vi "hcam_environment_monitor.vi"() -> ()   [LabVIEW 2020]
uses:
  <vilib>/Instr/_visa.llb/VISA Configure Serial Port (Instr).vi
panel:
  in  "INT 2":u8 caption="Brightness"
  in  "SEND INT 2":bool caption="Boolean"
  out "Humidity 2":string caption="Humidity"
  in  "Start 2":timestamp caption="Day Start" format="%<%H:%M>T"
  in  "End 2":timestamp caption="Day End" format="%<%H:%M>T"
  in  "SEND LED 2":bool caption="Boolean"
  in  "SEND RTC 2":bool caption="Boolean"
  in  "Color Box 2":u32(colorbox) caption="Color"
  out "Temp 2":string caption="Temp"
  in  "End":timestamp caption="Day End" format="%<%H:%M>T"
  in  "Start":timestamp caption="Day Start" format="%<%H:%M>T"
  in  "SEND LED":bool caption="Boolean"
  in  "Color Box":u32(colorbox) caption="Color"
  in  "SEND RTC":bool caption="Boolean"
  out "Humidity":string
  out "Temp":string
  in  "SEND INT":bool caption="Boolean"
  in  "INT":u8 caption="Brightness"
  out "Connected":bool
  out "Response":string
  in  "CONNECTION":bool
  out "Bytes Read":u32
  in  "VISA Resource":refnum<visa-resource-name>="COM1"
  # "--- Box 1 ---"
  # "--- Box 2 ---"
  # "Auto LED Timer"
  # "Auto LED Timer"
  # "Manual Color Control"
  # "Climate Readings"
  # "Manual Color Control"
  # "Climate Readings"
  # "Serial Monitor"
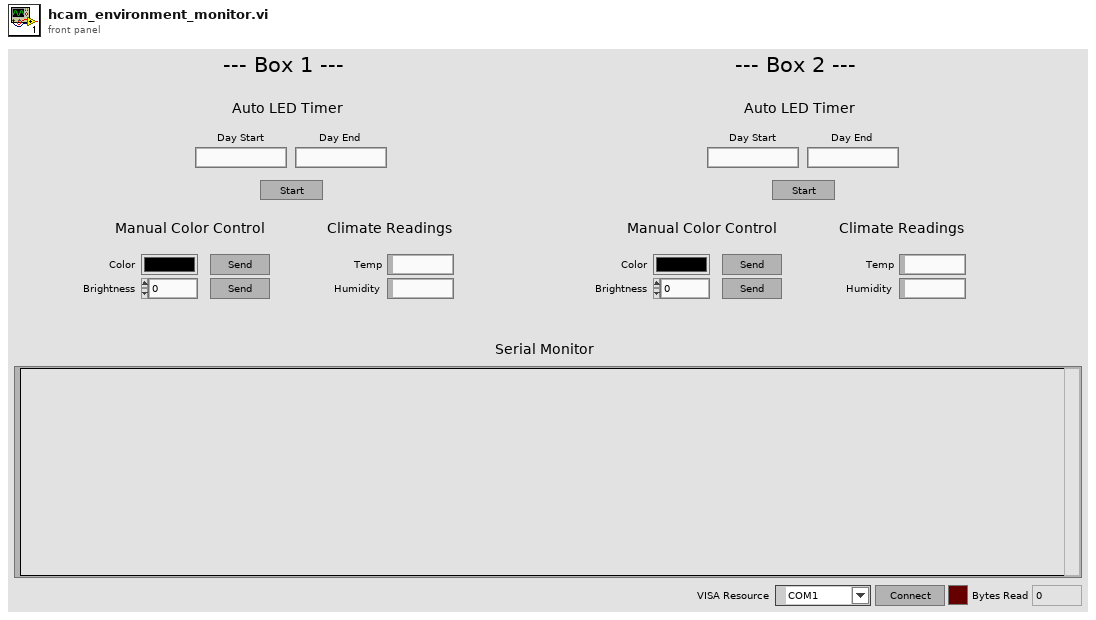
[diagram p1: front panel]
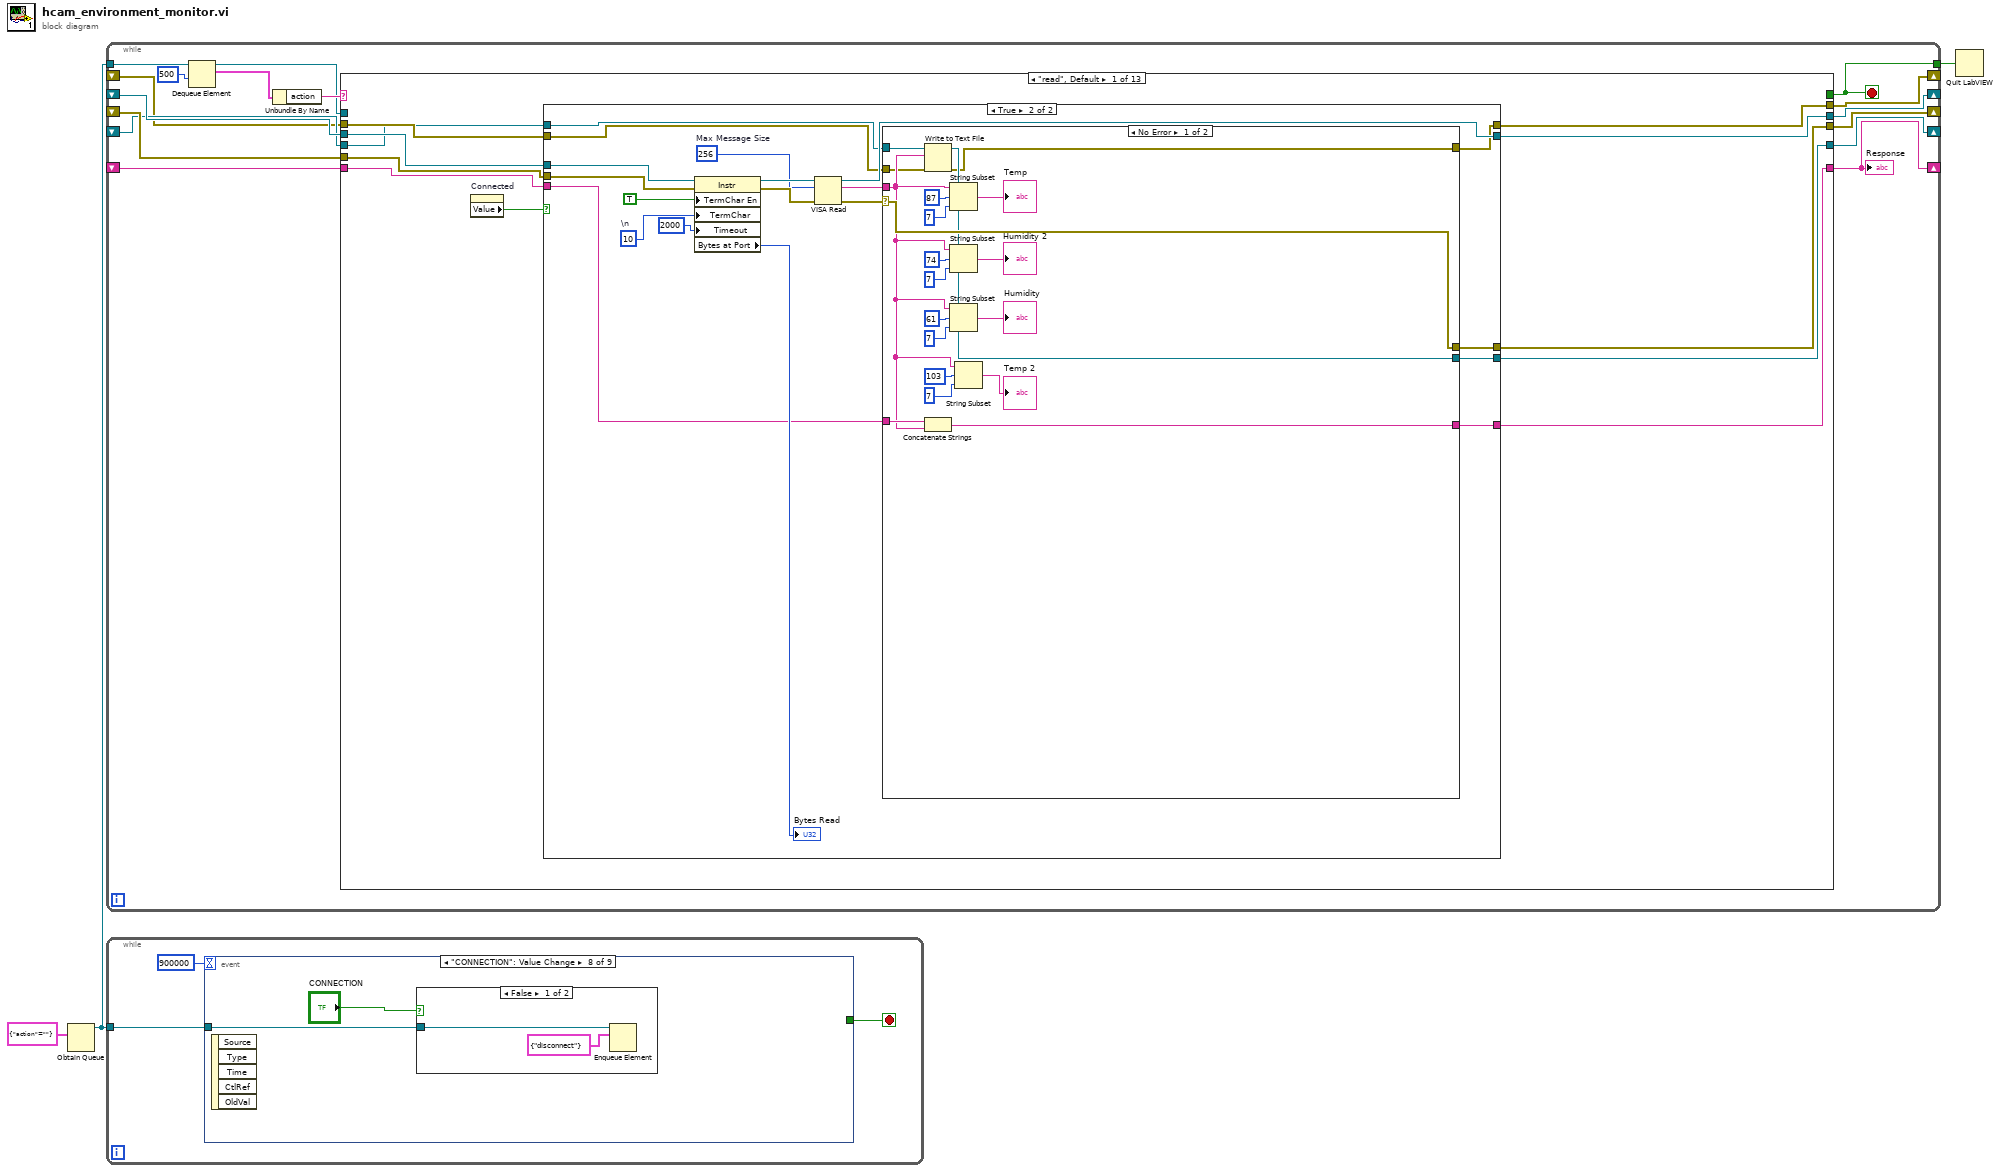
[diagram p0: block diagram]
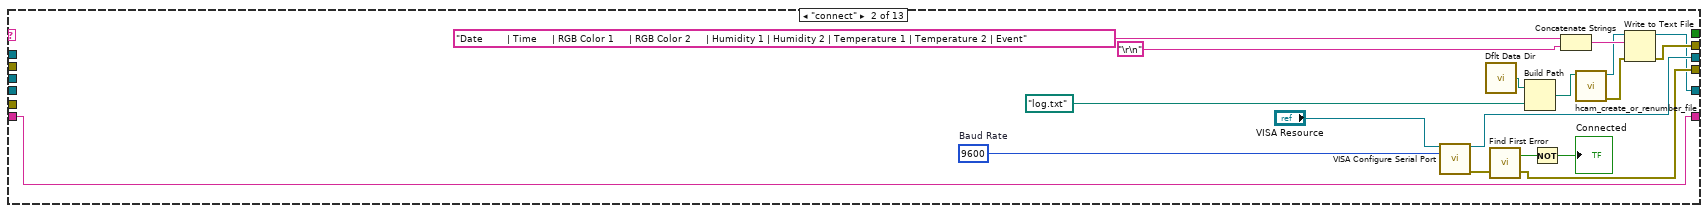
[diagram p4: hidden frame]
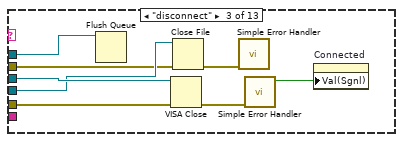
[diagram p5: hidden frame]
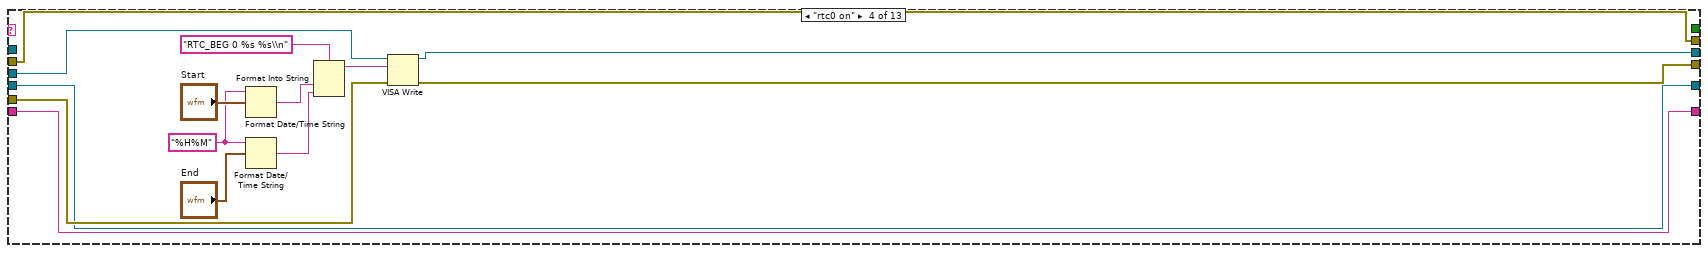
[diagram p6: hidden frame]
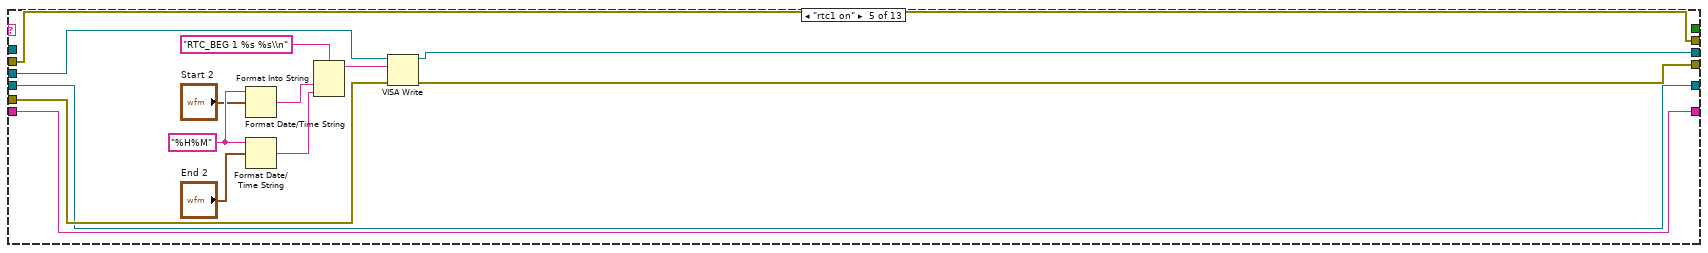
[diagram p7: hidden frame]
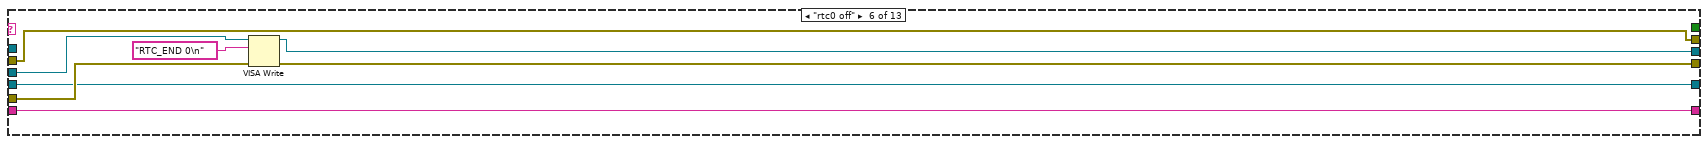
[diagram p8: hidden frame]
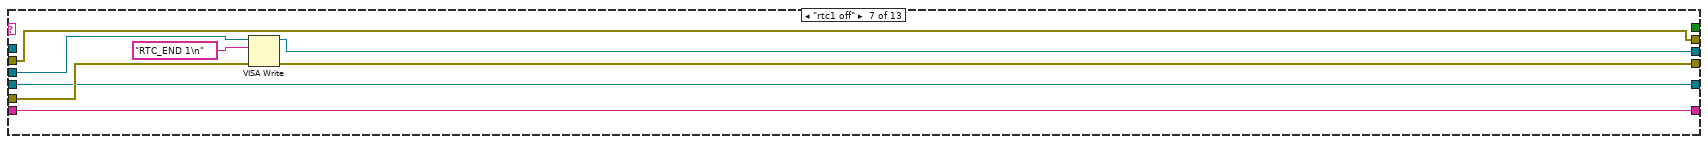
[diagram p9: hidden frame]
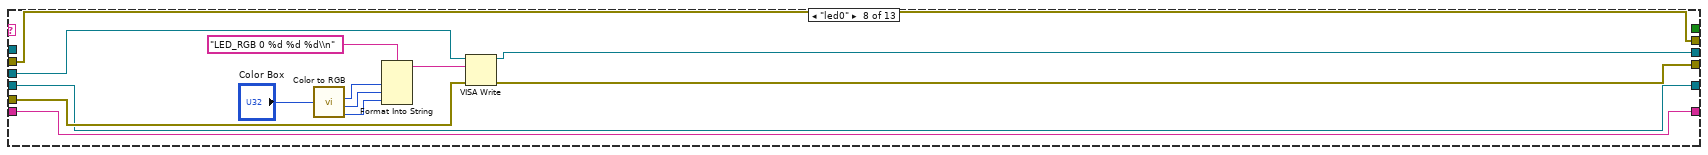
[diagram p10: hidden frame]
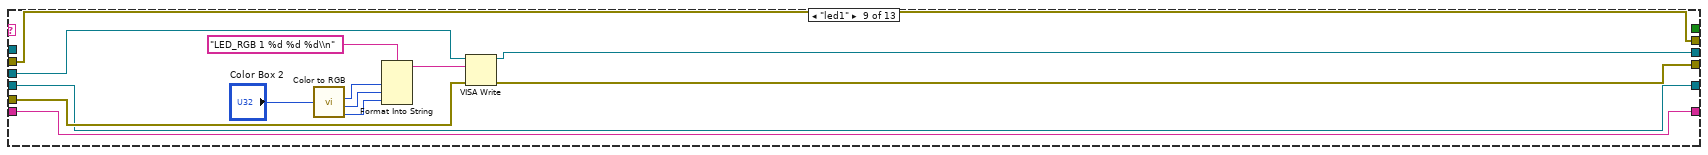
[diagram p11: hidden frame]
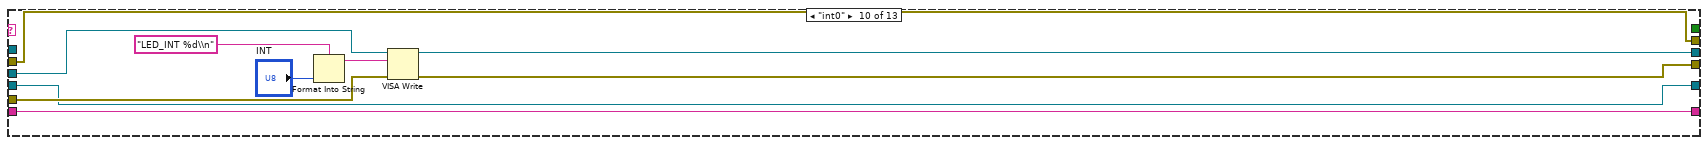
[diagram p12: hidden frame]
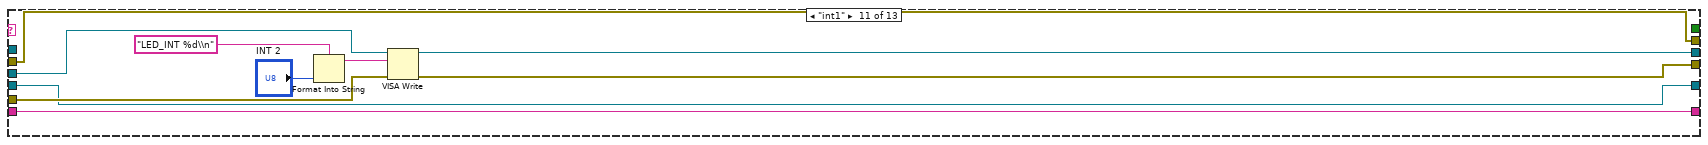
[diagram p13: hidden frame]
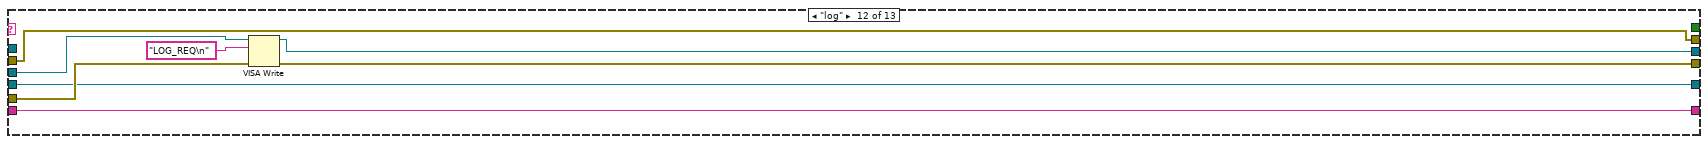
[diagram p14: hidden frame]
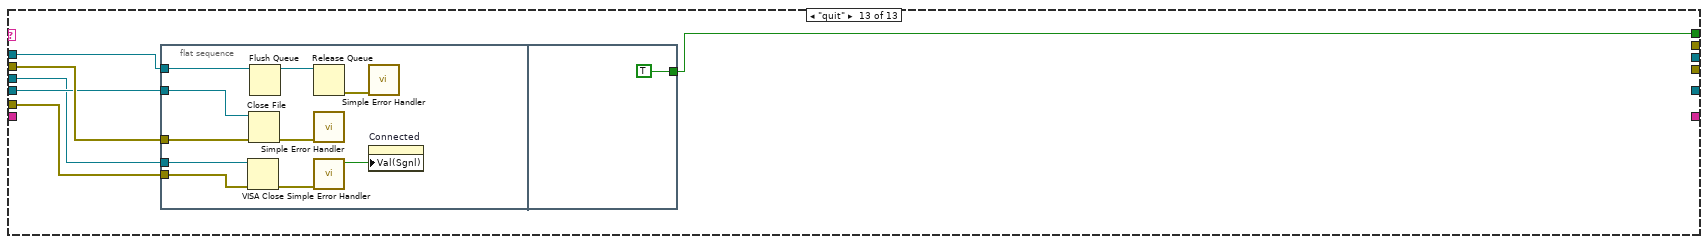
[diagram p15: hidden frame]
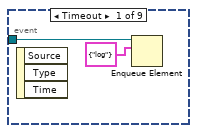
[diagram p16: hidden frame]
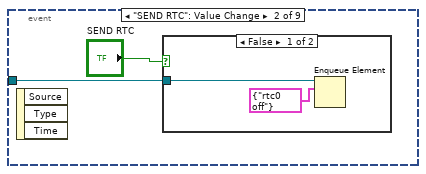
[diagram p17: hidden frame]
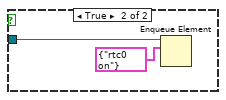
[diagram p18: hidden frame]
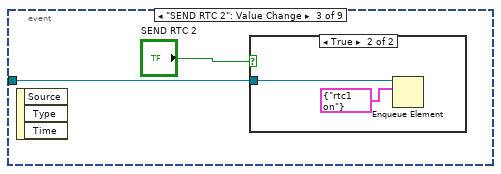
[diagram p19: hidden frame]
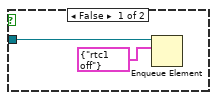
[diagram p20: hidden frame]
diagram:
  n1 = Obtain Queue(element data type=cluster{"action":string} {"action"=""}) -> (queue out=w2:refnum<queue>)  [unwired: 4 in, 2 out]
  n2 = while {
    tunnel: w2 -> [w19]
    shift-right: [w14] -> _
    shift-left: _ -> [w13]
    shift-right: [w12] -> _
    shift-left: _ -> [w11]
    shift-right: [w9] -> _
    shift-left: _ -> [w10]
    shift-right: [w6] -> _
    shift-left: _ -> [w8]
    shift-right: [w5] -> _
    shift-left: _ -> [w7]
    tunnel: [w4] -> w1
    stop <- w4 stop-if-true
    n3 = Dequeue Element(queue=w19, timeout in ms (-1)=500) -> (queue out=w15:refnum<queue>, element=w17:cluster{"action":string})  [unwired: 1 in, 2 out]
    n4 = Unbundle By Name(w17) -> ("action"=w16:string)
    n5 = case shown="\"read\", Default" w16 {
      tunnel: w15 -> [_ _ w95 _ _ _ _ _ _ _ _ _ w200]
      tunnel: [w24 w88 _ w104 w119 w133 w141 w152 w165 w175 w185 w192 _] -> w14
      tunnel: w13 -> [w30 _ w98 w105 w118 w134 w142 w153 w166 w176 w186 w193 w198]
      tunnel: [w28 w86 _ w102 w116 w131 w139 w150 w163 w172 w183 w194 _] -> w12
      tunnel: w11 -> [w29 _ w96 w103 w117 w132 w140 w151 w164 w173 w184 w195 w199]
      tunnel: [w26 w83 _ w101 w115 w130 w138 w149 w162 w171 w182 w196 _] -> w9
      tunnel: w10 -> [w27 w83 _ w101 w115 w130 w138 w149 w162 w171 w182 w196 _]
      tunnel: [w21 w79 _ w100 w114 w128 w136 w144 w157 w170 w180 w190 _] -> w6
      tunnel: [w20 w80 _ w99 w113 w127 w135 w143 w156 w169 w179 w189 _] -> w5
      tunnel: w8 -> [w22 _ w93 w100 w114 w128 w136 w144 w157 w170 w180 w190 w201]
      tunnel: w7 -> [w23 _ w92 w99 w113 w127 w135 w143 w156 w169 w179 w189 w202]
      tunnel: [_ _ _ _ _ _ _ _ _ _ _ _ w197] -> w4
      frame "read", Default {
        n6 = property on="Connected" class="Bool (strict)"() -> ("Value"=w25:bool)  [unwired: 2 in, 2 out]
        n7 = case shown="True" w25 {
          tunnel: w30 -> [_ w42]
          tunnel: w29 -> [_ w41]
          tunnel: [_ w36] -> w28
          tunnel: w27 -> [_ w38]
          tunnel: [_ w35] -> w26
          tunnel: [_ w40] -> w24
          tunnel: [_ w31] -> w20
          tunnel: [_ w32] -> w21
          tunnel: w23 -> [_ w34]
          tunnel: w22 -> [_ w33]
          frame False {
          }
          frame True {
            w46 = u32 256  # Max Message Size
            w44 = u8 10  # \n
            n8 = property class="Instr"(reference=w42, error in=w41, "TermChar En"=TRUE ("Message Based Settings:Termination Character Enable"), "TermChar"=w44, "Timeout"=u32 2000 ("General Settings:Timeout Value")) -> (reference out=w49:refnum<visa-resource-name>, error out=w48:errorcluster, "Bytes at Port"=→"Bytes Read":u32)
            n9 = VISA Read(VISA resource name=w49, byte count=w46, error in (no error)=w48) -> (VISA resource name out=w40:refnum<visa-resource-name>, read buffer=w37:string, error out=w39:errorcluster)  [unwired: 1 out]
            n10 = case shown="No Error" w39 {
              selector: w39 -> [w68 _]
              tunnel: w38 -> [w69 w72]
              tunnel: w37 -> [w54 _]
              tunnel: [w67 w72] -> w35
              tunnel: [w68 _] -> w36
              tunnel: w34 -> [w53 w71]
              tunnel: w33 -> [w52 w70]
              tunnel: [w51 w70] -> w32
              tunnel: [w50 w71] -> w31
              frame No Error {
                n11 = Write to Text File(file (use dialog)=w52, text=w54, error in=w53) -> (refnum out=w51:refnum<file>, error out=w50:errorcluster)  [unwired: 1 in, 1 out]
                n12 = Concatenate Strings(w69, w54) -> (w67:string)
                n13 = String Subset(string=w54, offset (0)=87, length (rest)=7) -> (substring=→"Temp":string)
                n14 = String Subset(string=w54, offset (0)=74, length (rest)=7) -> (substring=→"Humidity 2":string)
                n15 = String Subset(string=w54, offset (0)=61, length (rest)=7) -> (substring=→"Humidity":string)
                n16 = String Subset(string=w54, offset (0)=103, length (rest)=7) -> (substring=→"Temp 2":string)
              }
              frame Error {
              }
            }
          }
        }
      }
      frame "connect" {
        w89 = u32 9600  # Baud Rate
        n17 = call-poly "VISA Configure Serial Port"("VISA resource name"="VISA Resource", "baud rate (9600)"=w89) -> ("VISA resource name out"=w88:refnum<visa-resource-name>, "error out"=w87:errorcluster)  [unwired: 7 in, 5 out]
        n18 = call <vilib>:"Dflt Data Dir.vi"() -> ("App:Default Data Directory"=w82:path)
        n19 = call <vilib>:"Find First Error.vi"("error in (no error)"=w87) -> ("error out"=w86:errorcluster, "error?"=w85:bool)  [unwired: 3 in]
        n20 = Build Path(base path=w82, name or relative path=path "log.txt" ("default name")) -> (appended path=w75:path)
        n21 = Not(x=w85) -> (.not. x?=→"Connected":bool)
        n22 = Concatenate Strings("Date        | Time     | RGB Color 1     | RGB Color 2     | Humidity 1 | Humidity 2 | Temperature 1 | Temperature 2 | Event", "\r\n") -> (w76:string)
        n23 = call "hcam_create_or_renumber_file.vi"("file path"=w75) -> ("error out"=w73:errorcluster, "refnum out"=w74:refnum<file>)  [unwired: 9 in]
        n24 = Write to Text File(file (use dialog)=w74, text=w76, error in=w73) -> (refnum out=w79:refnum<file>, error out=w80:errorcluster)  [unwired: 1 in, 1 out]
      }
      frame "disconnect" {
        n25 = Flush Queue(queue=w95) -> ()  [unwired: 1 in, 3 out]
        n26 = VISA Close(VISA resource name=w98, error in (no error)=w96) -> (error out=w97:errorcluster)
        n27 = Close File(refnum=w93, error in=w92) -> (error out=w91:errorcluster)  [unwired: 1 out]
        n28 = call <vilib>:"Simple Error Handler.vi"("error in (no error)"=w91) -> ()  [unwired: 4 in, 5 out]
        n29 = call <vilib>:"Simple Error Handler.vi"("error in (no error)"=w97) -> ("error?"=w94:bool)  [unwired: 1 in, 7 out]
        n30 = property on="Connected" class="Bool (strict)"("Val(Sgnl)"=w94) -> ()  [unwired: 2 in, 2 out]
      }
      frame "rtc0 on" {
        w106 = "%H%M"
        n31 = Format Date/Time String(time format string (%c)=w106, seconds (now)="Start") -> (date/time string=w112:string)  [unwired: 1 in]
        n32 = Format Date/Time String(time format string (%c)=w106, seconds (now)="End") -> (date/time string=w111:string)  [unwired: 1 in]
        n33 = Format Into String(format string="RTC_BEG 0 %s %s\\n", w112, w111) -> (resulting string=w108:string)  [unwired: 2 in, 1 out]
        n34 = VISA Write(VISA resource name=w105, write buffer=w108, error in (no error)=w103) -> (VISA resource name out=w104:refnum<visa-resource-name>, error out=w102:errorcluster)  [unwired: 1 out]
      }
      frame "rtc1 on" {
        w124 = "%H%M"
        n35 = Format Date/Time String(time format string (%c)=w124, seconds (now)="Start 2") -> (date/time string=w122:string)  [unwired: 1 in]
        n36 = Format Date/Time String(time format string (%c)=w124, seconds (now)="End 2") -> (date/time string=w123:string)  [unwired: 1 in]
        n37 = Format Into String(format string="RTC_BEG 1 %s %s\\n", w122, w123) -> (resulting string=w125:string)  [unwired: 2 in, 1 out]
        n38 = VISA Write(VISA resource name=w118, write buffer=w125, error in (no error)=w117) -> (VISA resource name out=w119:refnum<visa-resource-name>, error out=w116:errorcluster)  [unwired: 1 out]
      }
      frame "rtc0 off" {
        n39 = VISA Write(VISA resource name=w134, write buffer="RTC_END 0\n" ("format string"), error in (no error)=w132) -> (VISA resource name out=w133:refnum<visa-resource-name>, error out=w131:errorcluster)  [unwired: 1 out]
      }
      frame "rtc1 off" {
        n40 = VISA Write(VISA resource name=w142, write buffer="RTC_END 1\n" ("format string"), error in (no error)=w140) -> (VISA resource name out=w141:refnum<visa-resource-name>, error out=w139:errorcluster)  [unwired: 1 out]
      }
      frame "led0" {
        n41 = call <vilib>:"Color to RGB.vi"("Color"="Color Box") -> ("R"=w147:u8, "G"=w146:u8, "B"=w145:u8)  [unwired: 1 out]
        n42 = Format Into String(format string="LED_RGB 0 %d %d %d\\n", w147, w146, w145) -> (resulting string=w154:string)  [unwired: 2 in, 1 out]
        n43 = VISA Write(VISA resource name=w153, write buffer=w154, error in (no error)=w151) -> (VISA resource name out=w152:refnum<visa-resource-name>, error out=w150:errorcluster)  [unwired: 1 out]
      }
      frame "led1" {
        n44 = call <vilib>:"Color to RGB.vi"("Color"="Color Box 2") -> ("R"=w160:u8, "G"=w159:u8, "B"=w158:u8)  [unwired: 1 out]
        n45 = Format Into String(format string="LED_RGB 1 %d %d %d\\n", w160, w159, w158) -> (resulting string=w167:string)  [unwired: 2 in, 1 out]
        n46 = VISA Write(VISA resource name=w166, write buffer=w167, error in (no error)=w164) -> (VISA resource name out=w165:refnum<visa-resource-name>, error out=w163:errorcluster)  [unwired: 1 out]
      }
      frame "int0" {
        n47 = Format Into String(format string="LED_INT %d\\n", "INT") -> (resulting string=w177:string)  [unwired: 2 in, 1 out]
        n48 = VISA Write(VISA resource name=w176, write buffer=w177, error in (no error)=w173) -> (VISA resource name out=w175:refnum<visa-resource-name>, error out=w172:errorcluster)  [unwired: 1 out]
      }
      frame "int1" {
        n49 = Format Into String(format string="LED_INT %d\\n", "INT 2") -> (resulting string=w187:string)  [unwired: 2 in, 1 out]
        n50 = VISA Write(VISA resource name=w186, write buffer=w187, error in (no error)=w184) -> (VISA resource name out=w185:refnum<visa-resource-name>, error out=w183:errorcluster)  [unwired: 1 out]
      }
      frame "log" {
        n51 = VISA Write(VISA resource name=w193, write buffer="LOG_REQ\n" ("format string"), error in (no error)=w195) -> (VISA resource name out=w192:refnum<visa-resource-name>, error out=w194:errorcluster)  [unwired: 1 out]
      }
      frame "quit" {
        n52 = flat-sequence {
          tunnel: w202 -> [w207]
          tunnel: w201 -> [w206]
          tunnel: w200 -> [w205]
          tunnel: w199 -> [w204]
          tunnel: w198 -> [w203]
          tunnel: [TRUE] -> w197
          frame #0 {
            n53 = VISA Close(VISA resource name=w203, error in (no error)=w204) -> (error out=w208:errorcluster)
            n54 = Close File(refnum=w206, error in=w207) -> (error out=w209:errorcluster)  [unwired: 1 out]
            n55 = Flush Queue(queue=w205) -> (queue out=w211:refnum<queue>)  [unwired: 1 in, 2 out]
            n56 = Release Queue(queue=w211) -> (error out=w212:errorcluster)  [unwired: 2 in, 2 out]
            n57 = call <vilib>:"Simple Error Handler.vi"("error in (no error)"=w209) -> ()  [unwired: 4 in, 5 out]
            n58 = call <vilib>:"Simple Error Handler.vi"("error in (no error)"=w208) -> ("error?"=w210:bool)  [unwired: 1 in, 7 out]
            n59 = call <vilib>:"Simple Error Handler.vi"("error in (no error)"=w212) -> ()  [unwired: 4 in, 5 out]
            n60 = property on="Connected" class="Bool (strict)"("Val(Sgnl)"=w210) -> ()  [unwired: 2 in, 2 out]
          }
          frame #1 {
          }
        }
      }
    }
    "Response" <- w9
  }
  n61 = while {
    tunnel: w2 -> [w216]
    stop <- w214 stop-if-true
    n62 = event shown="[7] \"CONNECTION\": Value Change" {
      selector: _ -> [_ _ _ _ _ _ _ _ _]
      dyn-events: _ -> [_ _ _ _ _ _ _ _ _]
      timeout: 900000 ("timeout in ms (-1)") -> [_ _ _ _ _ _ _ _ _]
      tunnel: w216 -> [w218 w219 w225 w231 w233 w235 w237 w240 w246]
      tunnel: [_ _ _ _ _ _ _ _ TRUE] -> w214
      event Timeout {
        n63 = event-data() -> ()  [unwired: 1 in, 3 out]
        n64 = Enqueue Element(queue=w218, element=cluster{"action":string} {"action"="log"}) -> ()  [unwired: 2 in, 3 out]
      }
      event "SEND RTC": Value Change {
        n65 = event-data() -> ()  [unwired: 1 in, 3 out]
        n66 = case shown="False" "SEND RTC" {
          tunnel: w219 -> [w221 w223]
          frame False {
            n67 = Enqueue Element(queue=w221, element=cluster{"action":string} {"action"="rtc0 off"}) -> ()  [unwired: 2 in, 3 out]
          }
          frame True {
            n68 = Enqueue Element(queue=w223, element=cluster{"action":string} {"action"="rtc0 on"}) -> ()  [unwired: 2 in, 3 out]
          }
        }
      }
      event "SEND RTC 2": Value Change {
        n69 = event-data() -> ()  [unwired: 1 in, 3 out]
        n70 = case shown="True" "SEND RTC 2" {
          tunnel: w225 -> [w227 w229]
          frame False {
            n71 = Enqueue Element(queue=w227, element=cluster{"action":string} {"action"="rtc1 off"}) -> ()  [unwired: 2 in, 3 out]
          }
          frame True {
            n72 = Enqueue Element(queue=w229, element=cluster{"action":string} {"action"="rtc1 on"}) -> ()  [unwired: 2 in, 3 out]
          }
        }
      }
      event "SEND LED": Value Change {
        n73 = event-data() -> ()  [unwired: 1 in, 3 out]
        n74 = Enqueue Element(queue=w231, element=cluster{"action":string} {"action"="led0"}) -> ()  [unwired: 2 in, 3 out]
      }
      event "SEND LED 2": Value Change {
        n75 = event-data() -> ()  [unwired: 1 in, 3 out]
        n76 = Enqueue Element(queue=w233, element=cluster{"action":string} {"action"="led1"}) -> ()  [unwired: 2 in, 3 out]
      }
      event "SEND INT": Value Change {
        n77 = event-data() -> ()  [unwired: 1 in, 6 out]
        n78 = Enqueue Element(queue=w235, element=cluster{"action":string} {"action"="int0"}) -> ()  [unwired: 2 in, 3 out]
      }
      event "SEND INT 2": Value Change {
        n79 = event-data() -> ()  [unwired: 1 in, 6 out]
        n80 = Enqueue Element(queue=w237, element=cluster{"action":string} {"action"="int1"}) -> ()  [unwired: 2 in, 3 out]
      }
      event "CONNECTION": Value Change {
        n81 = event-data() -> ()  [unwired: 1 in, 5 out]
        n82 = case shown="False" "CONNECTION" {
          tunnel: w240 -> [w241 w244]
          frame False {
            n83 = Enqueue Element(queue=w241, element=cluster{"action":string} {"action"="disconnect"}) -> ()  [unwired: 2 in, 3 out]
          }
          frame True {
            n84 = Enqueue Element(queue=w244, element=cluster{"action":string} {"action"="connect"}) -> ()  [unwired: 2 in, 3 out]
          }
        }
      }
      event Panel Close? {
        n85 = event-data() -> ()  [unwired: 1 in, 4 out]
        n86 = Enqueue Element(queue=w246, element=cluster{"action":string} {"action"="quit"}) -> ()  [unwired: 2 in, 3 out]
        n87 = event-data("Discard?"=TRUE) -> ()  [unwired: 1 in, 1 out]
      }
    }
  }
  n88 = Quit LabVIEW(quit? (T)=w1) -> ()
